vi "Set TWM Measurement.vi"(4 "status ref (none)":refnum<vi>, 7 "TWM Measurement properties":T1={"Sampling frequency (Hz)"=500000.0, "Record length (multiples of period)"=1000.0, "Signal amplitude (V)"=4.5, "Measurement frequency (Hz)"=1000.0, "Calculate RMS from samples"=FALSE, "Algorithm"="TWM-WFFT", "Measurement path"=""} {"Measurement frequency (Hz)" format="%#_3p"; "Record length (multiples of period)" format="%#_3p"; "Sampling frequency (Hz)" format="%#_3p"}, 8 "error in":errorcluster, 11 "TWM handle":i32) -> (0 "error out":errorcluster, 3 "TWM handle out":i32)   [LabVIEW 2020]
uses:
  Type definitions/Sampling properties.ctl
  external libraries/TWM-1.8.7.0-client/I64.vi
  external libraries/TWM-1.8.7.0-client/String.vi
  external libraries/TWM-1.8.7.0-client/EXT.vi
  external libraries/TWM-1.8.7.0-client/TWM Client.lvlib
  external libraries/TWM-1.8.7.0-client/infolib.lvlib
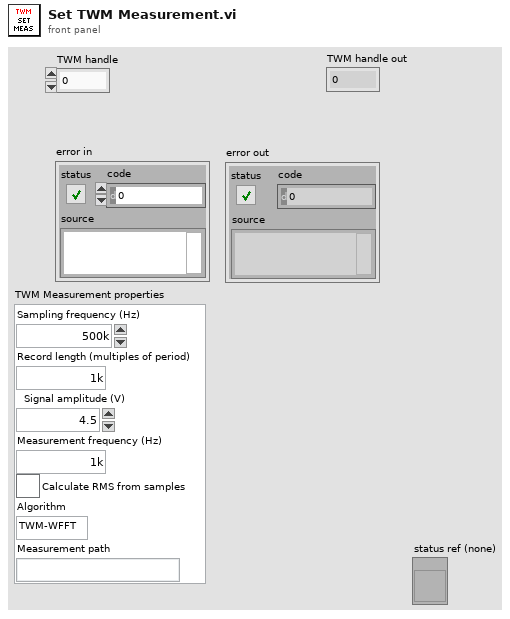
[diagram p1: front panel]
types:
  T1 = typedef "Sampling properties.ctl" = cluster{"Sampling frequency (Hz)":dbl, "Record length (multiples of period)":dbl, "Signal amplitude (V)":dbl, "Measurement frequency (Hz)":dbl, "Calculate RMS from samples":bool, "Algorithm":string, "Measurement path":string}
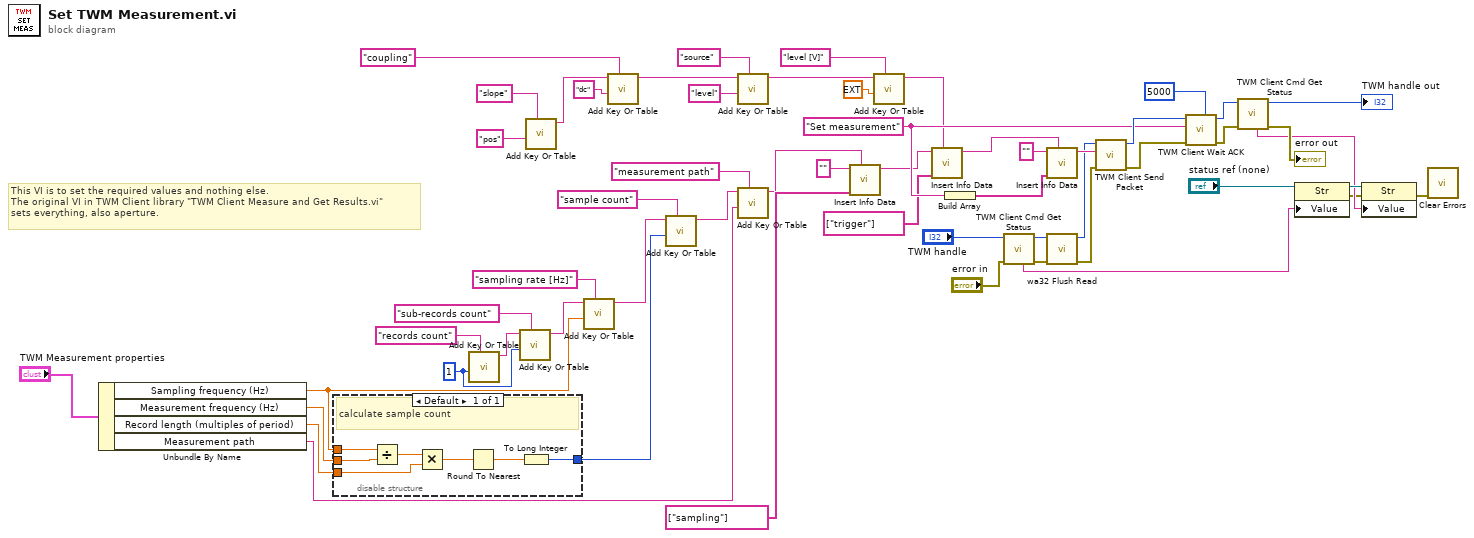
[diagram p0: block diagram]
diagram:
  w42 = 1 ("sub-records")
  w51 = "Set measurement" ("section name")
  # "This VI is to set the required values and nothing else.\nThe original VI in TWM Client library \"TWM Client Measure and Get Results.vi\"\nsets everything, also aperture."
  n1 = Unbundle By Name("TWM Measurement properties") -> ("Sampling frequency (Hz)"=w3:dbl, "Measurement frequency (Hz)"=w4:dbl, "Record length (multiples of period)"=w1:dbl, "Measurement path"=w2:string)
  n2 = disable-structure shown="Default" {
    disable-tunnel: w3 -> [w64]
    disable-tunnel: [w60] -> w9
    disable-tunnel: w1 -> [w59]
    disable-tunnel: w4 -> [w58]
    frame Enabled {
      # "calculate sample count"
      n3 = Divide(x=w64, y=w58) -> (x/y=w63:dbl)
      n4 = Multiply(x=w63, y=w59) -> (x*y=w62:dbl)
      n5 = Round To Nearest(number=w62) -> (nearest integer value=w61:dbl)
      n6 = To Long Integer(number=w61) -> (32bit integer=w60:i32)
    }
  }
  n7 = call-poly "Add Key Or Table.vi"("key description"="records count", "numeric"=w42) -> ("info data out"=w45:string)  [unwired: 8 in, 1 out]
  n8 = call-poly "Add Key Or Table.vi"("key description"="sub-records count", "numeric"=w42, "info data"=w45) -> ("info data out"=w40:string)  [unwired: 7 in, 1 out]
  n9 = call-poly "Add Key Or Table.vi"("key description"="slope", "string"="pos" ("key description")) -> ("info data out"=w25:string)  [unwired: 8 in, 1 out]
  n10 = call-poly "Add Key Or Table.vi"("key description"="sampling rate [Hz]", "numeric"=w3, "info data"=w40) -> ("info data out"=w39:string)  [unwired: 7 in, 1 out]
  n11 = call-poly "Add Key Or Table.vi"("key description"="coupling", "string"="dc" ("key description"), "info data"=w25) -> ("info data out"=w29:string)  [unwired: 7 in, 1 out]
  n12 = call-poly "Add Key Or Table.vi"("key description"="sample count", "numeric"=w9, "info data"=w39) -> ("info data out"=w8:string)  [unwired: 7 in, 1 out]
  n13 = call-poly "Add Key Or Table.vi"("key description"="source", "string"="level" ("key description"), "info data"=w29) -> ("info data out"=w31:string)  [unwired: 7 in, 1 out]
  n14 = call-poly "Add Key Or Table.vi"("key description"="measurement path", "string"=w2, "info data"=w8) -> ("info data out"=w7:string)  [unwired: 7 in, 1 out]
  n15 = call "Insert Info Data.vi"("info data to insert"=w7, "sections"=string[] ["sampling"], "info data"="") -> ("info data out"=w38:string)  [unwired: 7 in, 1 out]
  n16 = call-poly "Add Key Or Table.vi"("key description"="level [V]", "numeric"=ext 0.0, "info data"=w31) -> ("info data out"=w34:string)  [unwired: 7 in, 1 out]
  n17 = call "Insert Info Data.vi"("info data to insert"=w34, "sections"=string[] ["trigger"], "info data"=w38) -> ("info data out"=w37:string)  [unwired: 7 in, 1 out]
  n18 = Build Array(w51) -> (w56:string[])
  n19 = call "TWM Client Cmd Get Status.vi"("error in"="error in", "handle"="TWM handle") -> ("error out"=w13:errorcluster, "handle out"=w24:i32, "status string"=w22:string)  [unwired: 5 in, 2 out]
  n20 = call "Insert Info Data.vi"("info data to insert"=w37, "sections"=w56, "info data"="") -> ("info data out"=w57:string)  [unwired: 7 in, 1 out]
  n21 = call "wa32 Flush Read.vi"("error in"=w13, "handle"=w24) -> ("error out"=w50:errorcluster, "handle out"=w49:i32)  [unwired: 7 in, 1 out]
  n22 = call "TWM Client Send Packet.vi"("error in"=w50, "command string"=w57, "handle"=w49) -> ("error out"=w54:errorcluster, "handle out"=w53:i32)  [unwired: 7 in]
  n23 = call "TWM Client Wait ACK.vi"("timeout [ms] (3000)"=5000 ("timeout [ms] (1000)"), "error in"=w54, "command header"=w51, "handle"=w53) -> ("error out"=w20:errorcluster, "handle out"=w19:i32)  [unwired: 6 in]
  n24 = call "TWM Client Cmd Get Status.vi"("error in"=w20, "handle"=w19) -> ("error out"=→"error out":errorcluster, "handle out"=→"TWM handle out":i32, "status string"=w16:string)  [unwired: 5 in, 2 out]
  n25 = property class="Str"(reference="status ref (none)", "Value"=w22) -> (reference out=w21:refnum<vi>, error out=w14:errorcluster)  [unwired: 1 in]
  n26 = property class="Str"(reference=w21, error in=w14, "Value"=w16) -> (error out=w15:errorcluster)  [unwired: 1 out]
  n27 = call <vilib>:"Clear Errors.vi"("error in (no error)"=w15) -> ()  [unwired: 5 in, 2 out]
